vi "Query Instrument Temperature.vi"(8 "error in (no error)":errorcluster, 11 "U2000 in":refnum<class "U2000.lvclass">) -> (0 "error out":errorcluster, 2 "Temperature":dbl, 3 "U2000 out":refnum<class "U2000.lvclass">)   [LabVIEW 2020, in "U2000.lvclass"]
uses:
  U2000.lvclass
  C:/Sandbox/RF Bench/Source Code/WiSpry Test Framework/Instruments/Instrument.lvclass
  Instrument.lvclass/Instrument.ctl
  <instrlib>/Agilent U2000 Series/Agilent U2000 Series.lvlib
  Instrument.lvclass
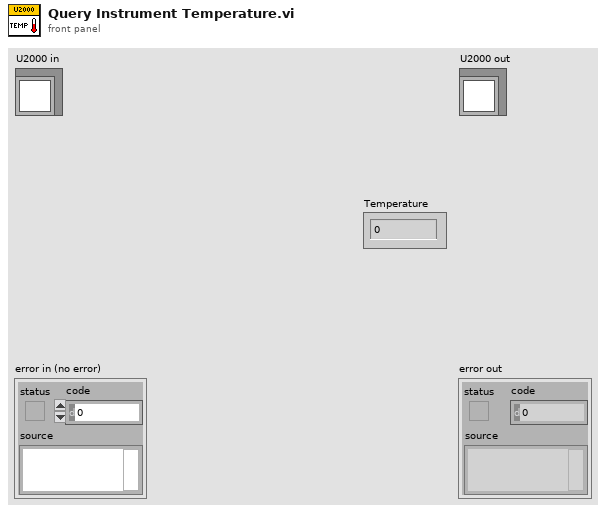
[diagram p1: front panel]
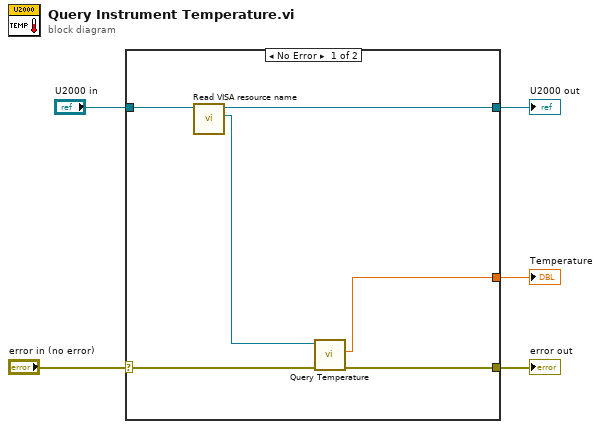
[diagram p0: block diagram]
diagram:
  n1 = case shown="No Error" "error in (no error)" {
    selector: "error in (no error)" -> [w11 w13]
    tunnel: [w10 w13] -> w4
    tunnel: [w8 w12] -> w3
    tunnel: "U2000 in" -> [w9 w12]
    tunnel: [w6 _] -> w1
    frame No Error {
      n2 = call "Read VISA resource name.vi"("Instrument in"=w9) -> ("VISA resource name"=w7:refnum<visa-resource-name>, "Instrument out"=w8:refnum<class "U2000.lvclass">)  [unwired: 9 in]
      n3 = call <instrlib>:"Query Temperature.vi"("error in (no error)"=w11, "VISA resource name"=w7) -> ("error out"=w10:errorcluster, "Temperature"=w6:dbl)  [unwired: 7 in, 1 out]
    }
    frame Error {
    }
  }
  "error out" <- w4
  "U2000 out" <- w3
  "Temperature" <- w1
